vi "Vote.vi"(9 "VoterInfo":T1, 10 "VoterID":i32, 11 "map in":map{i32, T1}(c390)) -> (3 "map out":map{i32, T1}(c390))   [LabVIEW 2019]
doc: "Update the voter registration map with the vote from the voter (connection)."
uses:
  SubVIs/Voter Info.ctl
  <vilib>/Utility/miscctls.llb/LVMapReplaceAction.ctl
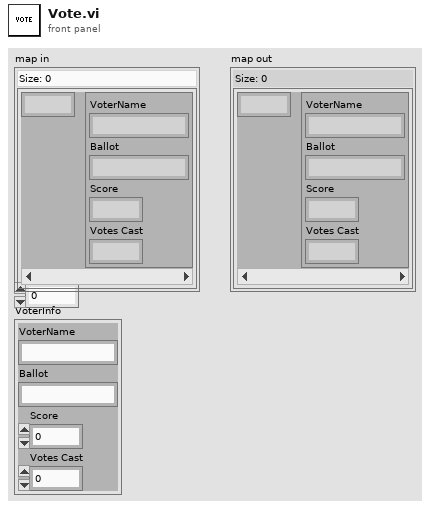
[diagram p1: front panel]
types:
  T1 = typedef "Voter Info.ctl" = cluster{"VoterName":string, "Ballot":string, "Score":i32, "Votes Cast":i32}
  T2 = typedef "LVMapReplaceAction.ctl" = enum32{"Modify Entry only if found", "Add or Modify Entry", "Delete Entry"}
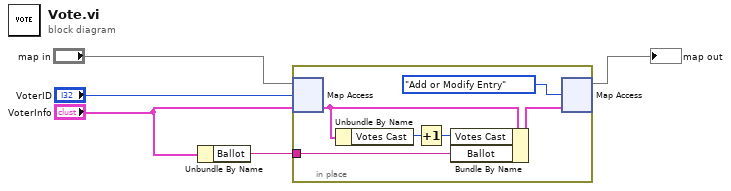
[diagram p0: block diagram]
diagram:
  n1 = Unbundle By Name("VoterInfo") -> ("Ballot"=w1:string)
  n2 = in-place {
    in-place-border: w1 -> [w11]
    n3 = in-place-map #1("map in", "VoterID", "VoterInfo") -> (w8:T1)  [unwired: 1 out]
    n4 = Unbundle By Name(w8) -> ("Votes Cast"=w7:i32)
    n5 = Increment(x=w7) -> (x+1=w6:i32)
    n6 = Bundle By Name(cluster=w8, "Votes Cast"=w6, "Ballot"=w11) -> (w10:T1)
    n7 = in-place-map #1(w10, LVMapReplaceAction."Add or Modify Entry" ("action")) -> (→"map out":map{i32, T1})  [unwired: 2 out]
  }
